vi "0_PlanVirtualStave.vi"(0 "Tape Type":T1=enum."Left stereo", 2 "Stave Locking Points [mm]":dbl[][](array[numeric])=[[0.0, 0.0, 0.0], [280.05, 0.0, 0.0], [574.05, 0.0, 0.0], [868.05, 0.0, 0.0], [1162.05, 0.0, 0.0]], 3 "Code path":path=path "C:/Users/sciollalab/Documents/Brandeis-BNL/LabVIEW_Codes/BNL_ThermomechanicalStave", 5 "Module fiducial marker":T3, 7 "Sensor Pattern":T2=enum."ATLAS12", 9 "N Modules":i32=13, 11 "Working height [mm]":dbl, 12 "error in (no error)":errorcluster, 13 "Stereo Angle [mrad]":dbl=26.0 format="%#_13g") -> (4 "Stave Basis: Coordinates of Fiducials on Modules":dbl[][](array[numeric])=[[-7.689999999999998, -113.212, 0.0], [87.79, -113.212, 0.0], [87.79, -16.13199999999999, 0.0], [-7.689999999999998, -16.13199999999999, 0.0], [90.31, -113.212, 0.0], [185.79000000000002, -113.212, 0.0], [185.79000000000002, -16.13199999999999, 0.0], [90.31, -16.13199999999999, 0.0], [188.31, -113.212, 0.0], [283.79, -113.212, 0.0], [283.79, -16.13199999999999, 0.0], [188.31, -16.13199999999999, 0.0], [286.31, -113.212, 0.0], [381.79, -113.212, 0.0], [381.79, -16.13199999999999, 0.0], [286.31, -16.13199999999999, 0.0], [384.31, -113.212, 0.0], [479.79, -113.212, 0.0], [479.79, -16.13199999999999, 0.0], [384.31, -16.13199999999999, 0.0], [482.30999999999995, -113.212, 0.0], [577.79, -113.212, 0.0], [577.79, -16.13199999999999, 0.0], [482.30999999999995, -16.13199999999999, 0.0], [580.31, -113.212, 0.0], [675.79, -113.212, 0.0], [675.79, -16.13199999999999, 0.0], [580.31, -16.13199999999999, 0.0], [678.31, -113.212, 0.0], [773.79, -113.212, 0.0], [773.79, -16.13199999999999, 0.0], [678.31, -16.13199999999999, 0.0], [776.31, -113.212, 0.0], [871.79, -113.212, 0.0], [871.79, -16.13199999999999, 0.0], [776.31, -16.13199999999999, 0.0], [874.31, -113.212, 0.0], [969.79, -113.212, 0.0], [969.79, -16.13199999999999, 0.0], [874.31, -16.13199999999999, 0.0], [972.31, -113.212, 0.0], [1067.79, -113.212, 0.0], [1067.79, -16.13199999999999, 0.0], [972.31, -16.13199999999999, 0.0], [1070.31, -113.212, 0.0], [1165.79, -113.212, 0.0], [1165.79, -16.13199999999999, 0.0], [1070.31, -16.13199999999999, 0.0], [1168.31, -113.212, 0.0], [1263.79, -113.212, 0.0], [1263.79, -16.13199999999999, 0.0], [1168.31, -16.13199999999999, 0.0]], 14 "error out":errorcluster, 15 "Module fiducials in the Stave's basis":T4(graph)=[{"Generated List of Module Coordinates"=[0.0, 280.05, 574.05, 868.05, 1162.05], "Generated List of Module Coordinates"=[0.0, 0.0, 0.0, 0.0, 0.0]}, {"Generated List of Module Coordinates"=[-7.689999999999998, 87.79, 87.79, -7.689999999999998, 90.31, 185.79000000000002, 185.79000000000002, 90.31, 188.31, 283.79, 283.79, 188.31, 286.31, 381.79, 381.79, 286.31, 384.31, 479.79, 479.79, 384.31, 482.30999999999995, 577.79, 577.79, 482.30999999999995, 580.31, 675.79, 675.79, 580.31, 678.31, 773.79, 773.79, 678.31, 776.31, 871.79, 871.79, 776.31, 874.31, 969.79, 969.79, 874.31, 972.31, 1067.79, 1067.79, 972.31, 1070.31, 1165.79, 1165.79, 1070.31, 1168.31, 1263.79, 1263.79, 1168.31], "Generated List of Module Coordinates"=[-113.212, -113.212, -16.13199999999999, -16.13199999999999, -113.212, -113.212, -16.13199999999999, -16.13199999999999, -113.212, -113.212, -16.13199999999999, -16.13199999999999, -113.212, -113.212, -16.13199999999999, -16.13199999999999, -113.212, -113.212, -16.13199999999999, -16.13199999999999, -113.212, -113.212, -16.13199999999999, -16.13199999999999, -113.212, -113.212, -16.13199999999999, -16.13199999999999, -113.212, -113.212, -16.13199999999999, -16.13199999999999, -113.212, -113.212, -16.13199999999999, -16.13199999999999, -113.212, -113.212, -16.13199999999999, -16.13199999999999, -113.212, -113.212, -16.13199999999999, -16.13199999999999, -113.212, -113.212, -16.13199999999999, -16.13199999999999, -113.212, -113.212, -16.13199999999999, -16.13199999999999]}, {"Generated List of Module Coordinates"=[40.050000000000004, 138.05, 236.05, 334.05, 432.05, 530.05, 628.05, 726.05, 824.05, 922.05, 1020.05, 1118.05, 1216.05], "Generated List of Module Coordinates"=[-64.672, -64.672, -64.672, -64.672, -64.672, -64.672, -64.672, -64.672, -64.672, -64.672, -64.672, -64.672, -64.672]}])   [LabVIEW 2016]
uses:
  Utils/Controls/All_Enums/Enum_TypeDef_FidMarkers.ctl
  Utils/Controls/All_Enums/Enum_TypeDef_Sensors.ctl
  Utils/Controls/All_Enums/Enum_TypeDef_TapeType.ctl
panel:
  in  "Intermodule pitch [mm]":dbl=98.0
  out "Module height [mm]":dbl=97.54
  out "Module width [mm]":dbl=97.54
  in  "Tab Control":enum32{"Stave Configuration", "Error reporting"}(tab)
  out "Stave orientation":bool=TRUE
  in  "Module centre [mm]":T5
  # "PLAN VIRTUAL STAVE Brandeis University - Brookhaven National Laboratory * ATLAS Phase II Inner Tracker Upgrade"
  # "F"
  # "F"
  # "F"
  # "F"
  # "This VI calculates the positions of all fiducials, \"F\",  on the modules on the stave. Supply the bus tape type, sensor design, desired fiducial marker, and number of modules."
  # "F"
  # "F"
  # "F"
  # "F"
  # "Provided by Camera Calibration:"
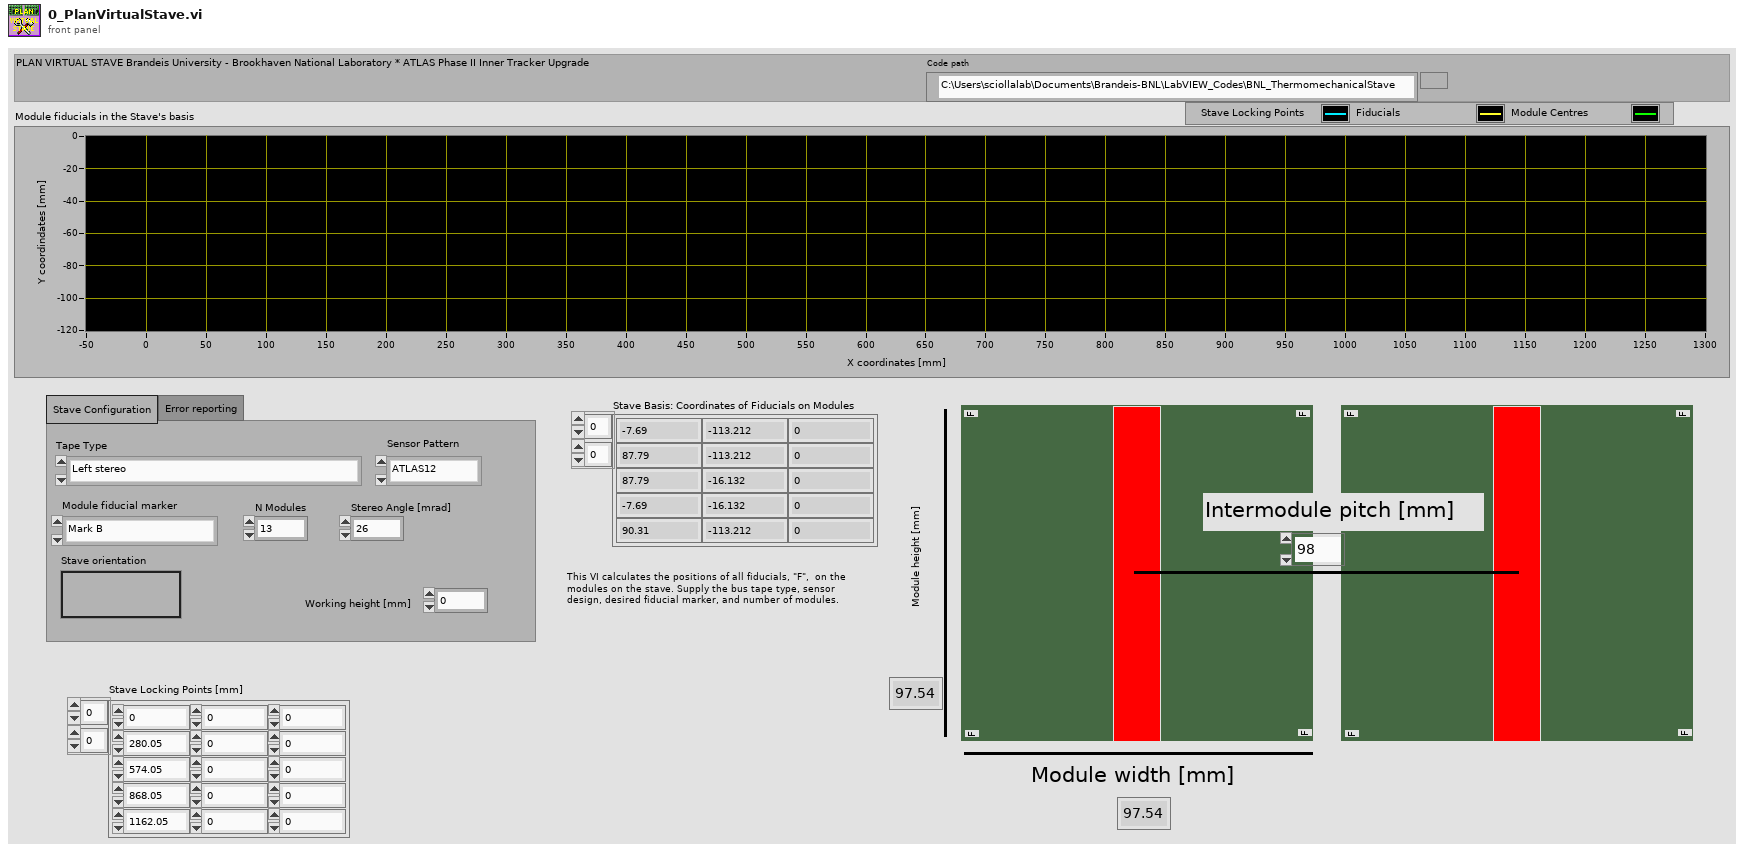
[diagram p1: front panel]
types:
  T1 = typedef "Enum_TypeDef_TapeType.ctl" = enum16{"Right stereo", "Left stereo", "Stereo (Sutcliffe NP49-01-100 01-Mar-16)", "Axial (Sutcliffe NP49-01-100 01-Mar-16)"}
  T2 = typedef "Enum_TypeDef_Sensors.ctl" = enum16{"ATLAS07", "ATLAS12", "ATLAS12Slim", "ATLAS17LS"}
  T3 = typedef "Enum_TypeDef_FidMarkers.ctl" = enum16{"Mark B", "Mark C", "Bias Ring Corner", "Mark I (Slim/17)", "Mark E (Slim/17)", "Mark F (Slim/17)", "Mark G (Slim/17)", "Mark A (12)", "Kapton Spacers"}
  T4 = cluster{"Generated List of Module Coordinates":dbl[], "Generated List of Module Coordinates":dbl[]}[]
  T5 = cluster{"X [mm]":dbl, "Y [mm]":dbl, "Z [mm]":dbl}
  T6 = enum8{"Enabled", "Disabled", "Disabled and Grayed Out"}
  T7 = cluster{"Stave Locking Points [mm]":dbl[], "Stave Locking Points [mm]":dbl[]}
  T8 = cluster{"Generated List of Module Coordinates":dbl[], "Generated List of Module Coordinates":dbl[]}
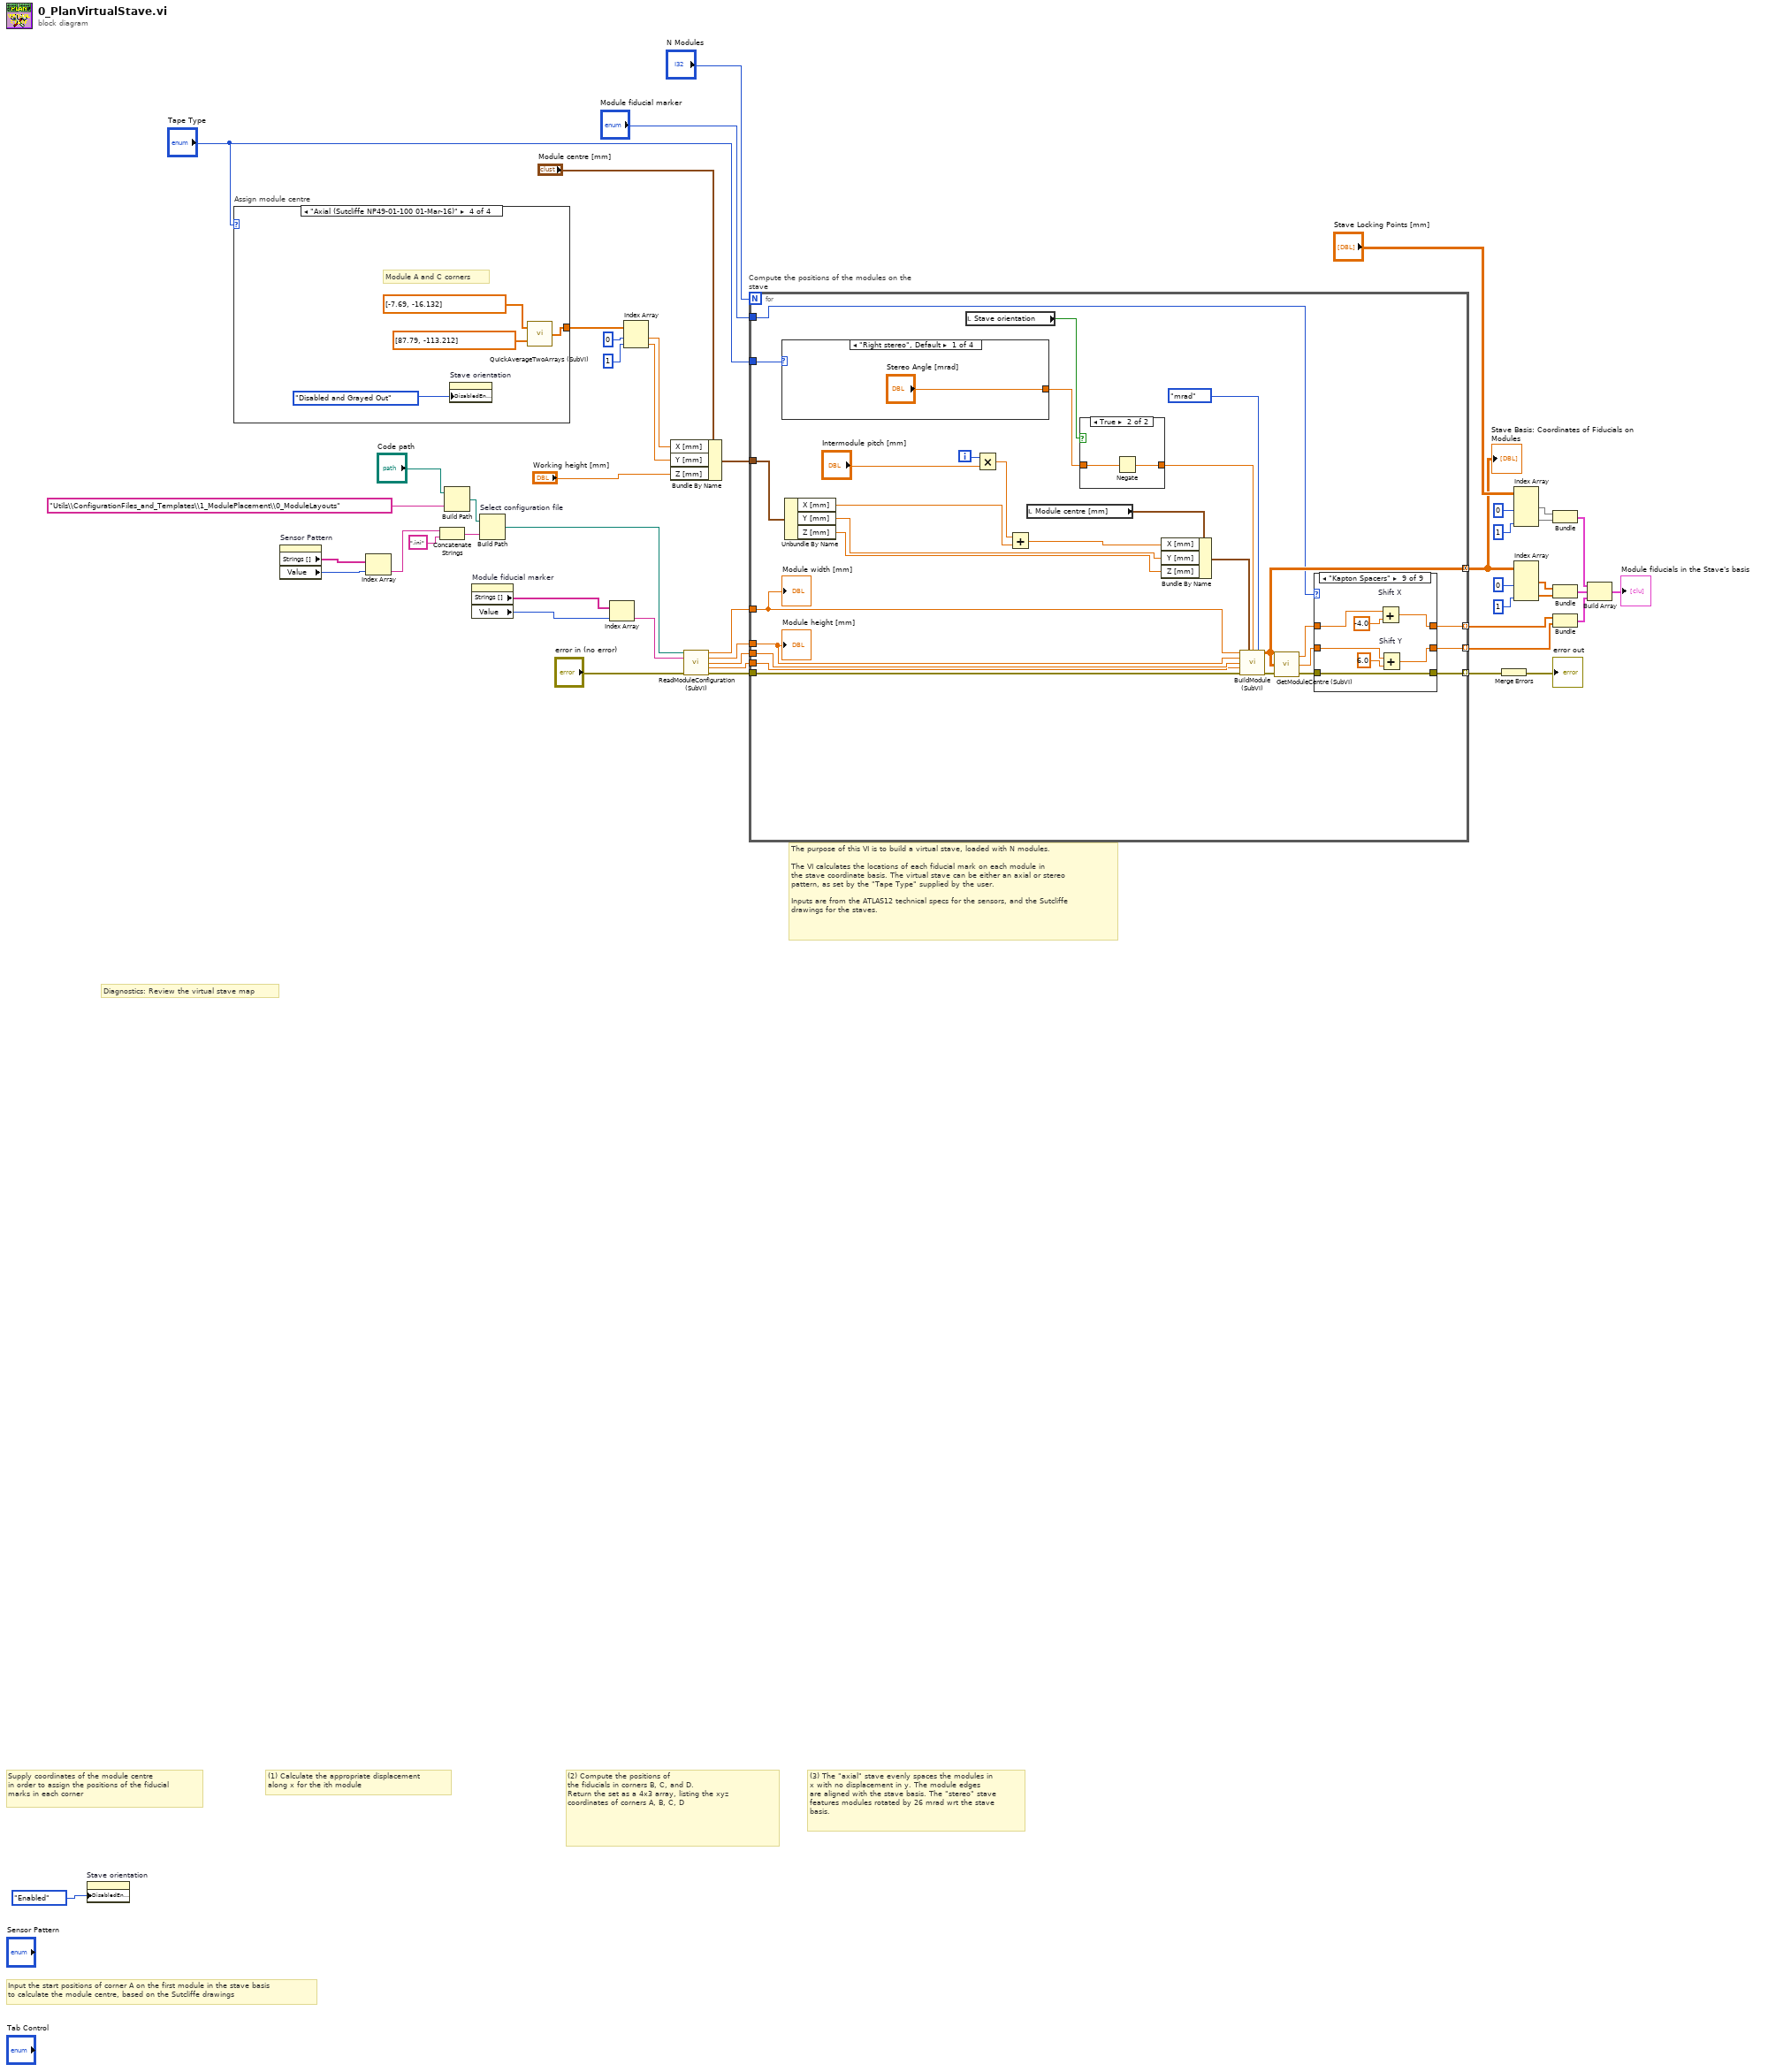
[diagram p0: block diagram]
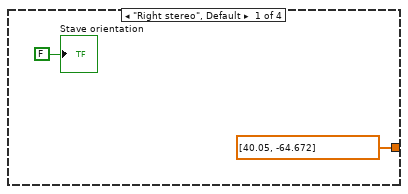
[diagram p2: hidden frame]
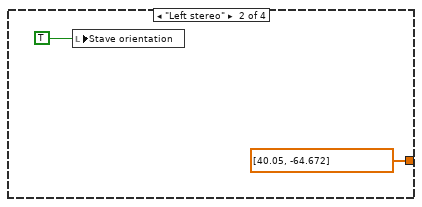
[diagram p3: hidden frame]
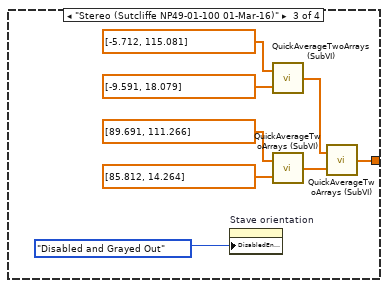
[diagram p4: hidden frame]
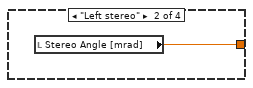
[diagram p14: hidden frame]
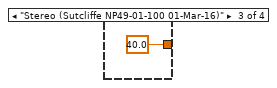
[diagram p15: hidden frame]
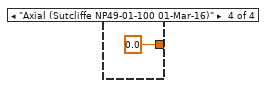
[diagram p16: hidden frame]
diagram:
  # "(1) Calculate the appropriate displacement \nalong x for the ith module"
  # "(3) The \"axial\" stave evenly spaces the modules in \nx with no displacement in y. The module edges \nare aligned with the stave basis. The \"stereo\" stave \nfeatures modules rotated by 26 mrad wrt the stave\nbasis."
  # "(2) Compute the positions of \nthe fiducials in corners B, C, and D. \nReturn the set as a 4x3 array, listing the xyz coordinates of corners A, B, C, D"
  # "Supply coordinates of the module centre \nin order to assign the positions of the fiducial \nmarks in each corner"
  # "Diagnostics: Review the virtual stave map"
  # "Input the start positions of corner A on the first module in the stave basis\nto calculate the module centre, based on the Sutcliffe drawings"
  # "The purpose of this VI is to build a virtual stave, loaded with N modules.\n\nThe VI calculates the locations of each fiducial mark on each module in \nthe stave coordinate basis. The virtual stave can be either an axial or stereo \npattern, as set by the \"Tape Type\" supplied by the user.\n\nInputs are from the ATLAS12 technical specs for the sensors, and the Sutcliffe\ndrawings for the staves."
  n1 = property on="Stave orientation" class="Bool"("DisabledEnum"=T6."Enabled" ("Disabled")) -> ()  [unwired: 2 in, 2 out]
  n2 = case "Assign module centre" shown="\"Axial (Sutcliffe NP49-01-100 01-Mar-16)\"" "Tape Type" {
    tunnel: [dbl[] [40.05, -64.672] ("Average of A and B") dbl[] [40.05, -64.672] ("Average of A and B") w54 w62] -> w27
    frame "Right stereo", Default {
      "Stave orientation" <- FALSE ("Stave orientation")
    }
    frame "Left stereo" {
      n3 = local write "Stave orientation"(TRUE ("Stave orientation")) -> ()
    }
    frame "Stereo (Sutcliffe NP49-01-100 01-Mar-16)" {
      n4 = property on="Stave orientation" class="Bool"("DisabledEnum"=T6."Disabled and Grayed Out" ("Disabled")) -> ()  [unwired: 2 in, 2 out]
      n5 = call "QuickAverageTwoArrays (SubVI).vi"("B"=dbl[] [-9.591, 18.079], "A"=dbl[] [-5.712, 115.081]) -> ("Average of A and B"=w59:dbl[])
      n6 = call "QuickAverageTwoArrays (SubVI).vi"("B"=dbl[] [85.812, 14.264], "A"=dbl[] [89.691, 111.266]) -> ("Average of A and B"=w60:dbl[])
      n7 = call "QuickAverageTwoArrays (SubVI).vi"("B"=w60, "A"=w59) -> ("Average of A and B"=w54:dbl[])
    }
    frame "Axial (Sutcliffe NP49-01-100 01-Mar-16)" {
      # "Module A and C corners"
      n8 = property on="Stave orientation" class="Bool"("DisabledEnum"=T6."Disabled and Grayed Out" ("Disabled")) -> ()  [unwired: 2 in, 2 out]
      n9 = call "QuickAverageTwoArrays (SubVI).vi"("B"=dbl[] [87.79, -113.212], "A"=dbl[] [-7.69, -16.132]) -> ("Average of A and B"=w62:dbl[])
    }
  }
  n10 = property on="Sensor Pattern" class="Enum (strict)"() -> ("Strings []"=w7:string[], "Value"=w6:T2)  [unwired: 2 in, 2 out]
  n11 = Index Array(array=w7, index=w6) -> (element=w5:string)
  n12 = Concatenate Strings(w5, ".ini" ("string")) -> (w3:string)
  n13 = Build Path(base path="Code path", name or relative path="Utils\\ConfigurationFiles_and_Templates\\1_ModulePlacement\\0_ModuleLayouts") -> (appended path=w2:path)
  n14 = property on="Module fiducial marker" class="Enum (strict)"() -> ("Strings []"=w10:string[], "Value"=w9:T3)  [unwired: 2 in, 2 out]
  n15 = Build Path "Select configuration file"(base path=w2, name or relative path=w3) -> (appended path=w1:path)
  n16 = Index Array(array=w10, index=w9) -> (element=w8:string)
  n17 = Index Array(array=w27, index #1=0 ("index"), index #2=1 ("index")) -> (element #1=w30:dbl, element #2=w28:dbl)
  n18 = Bundle By Name(cluster="Module centre [mm]", "X [mm]"=w30, "Y [mm]"=w28, "Z [mm]"="Working height [mm]") -> (w44:T5)
  n19 = call "ReadModuleConfiguration (SubVI).vi"("Module configuration file path"=w1, "Fiducial Mark"=w8, "error in (no error)"="error in (no error)") -> ("Width [mm]"=w18:dbl, "Height [mm]"=w17:dbl, "Lx"=w16:dbl, "Ly"=w15:dbl, "error out"=w19:errorcluster)  [unwired: 6 in, 2 out]
  n20 = for "Compute the positions of the modules on the stave" {
    N: "N Modules" -> [_]
    tunnel: w44 -> [w87]
    tunnel: [w84] -> w12 mode=concatenating
    tunnel: [w70] -> w36 mode=indexing
    tunnel: [w68] -> w26 mode=indexing
    tunnel: [w66] -> w24 mode=indexing
    tunnel: w19 -> [w82]
    tunnel: w18 -> [w79]
    tunnel: w17 -> [w78]
    tunnel: w16 -> [w81]
    tunnel: w15 -> [w80]
    tunnel: "Tape Type" -> [w75]
    tunnel: "Module fiducial marker" -> [w65]
    i -> [w93]
    n21 = case shown="\"Right stereo\", Default" w75 {
      tunnel: ["Stereo Angle [mrad]" w129 40.0 ("Stereo Angle [mrad]") 0.0 ("Angle")] -> w73
      frame "Right stereo", Default {
      }
      frame "Left stereo" {
        n22 = local read "Stereo Angle [mrad]"() -> (w129:dbl)
      }
      frame "Stereo (Sutcliffe NP49-01-100 01-Mar-16)" {
      }
      frame "Axial (Sutcliffe NP49-01-100 01-Mar-16)" {
      }
    }
    n23 = Unbundle By Name(w87) -> ("X [mm]"=w92:dbl, "Y [mm]"=w90:dbl, "Z [mm]"=w88:dbl)
    n24 = local read "Stave orientation"() -> (w74:bool)
    n25 = Multiply(x=w93, y="Intermodule pitch [mm]") -> (x*y=w91:dbl)
    n26 = Add(x=w91, y=w92) -> (x+y=w89:dbl)
    n27 = local read "Module centre [mm]"() -> (w76:T5)
    n28 = case shown="True" w74 {
      tunnel: w73 -> [w125 w127]
      tunnel: [w125 w126] -> w72
      frame False {
      }
      frame True {
        n29 = Negate(x=w127) -> (-x=w126:dbl)
      }
    }
    n30 = Bundle By Name(cluster=w76, "X [mm]"=w89, "Y [mm]"=w90, "Z [mm]"=w88) -> (w86:T5)
    n31 = call "BuildModule (SubVI).vi"("Module width[mm]"=w79, "Module Centre [mm]"=w86, "Angle"=w72, "Units"=enum16{"mrad", "Radians", "Degrees"}."mrad", "Module height [mm]"=w78, "x to fiducial [um]"=w81, "y to fiducial [um]"=w80, "error in (no error)"=w82) -> ("Generated List of Module Coordinates"=w84:dbl[][], "error out"=w83:errorcluster)  [unwired: 6 in]
    n32 = call "GetModuleCentre (SubVI).vi"("error in (no error)"=w83, "4x3 Array of Fiducial Coordinates"=w84) -> ("error out"=w67:errorcluster, "y, centre"=w69:dbl, "x, centre"=w71:dbl)  [unwired: 1 in]
    n33 = case shown="\"Kapton Spacers\"" w65 {
      tunnel: w71 -> [w96 w99 w101 w105 w107 w110 w113 w117 w121]
      tunnel: [w96 w99 w101 w105 w107 w110 w113 w117 w120] -> w70
      tunnel: w69 -> [w95 w98 w100 w104 w106 w109 w112 w116 w124]
      tunnel: [w95 w98 w100 w104 w106 w109 w112 w116 w119] -> w68
      tunnel: w67 -> [w94 w97 w102 w103 w108 w111 w114 w115 w118]
      tunnel: [w94 w97 w102 w103 w108 w111 w114 w115 w118] -> w66
      frame "Mark B", Default {
      }
      frame "Mark C" {
      }
      frame "Bias Ring Corner" {
      }
      frame "Mark I (Slim/17)" {
      }
      frame "Mark E (Slim/17)" {
      }
      frame "Mark F (Slim/17)" {
      }
      frame "Mark G (Slim/17)" {
      }
      frame "Mark A (12)" {
      }
      frame "Kapton Spacers" {
        n34 = Add "Shift X"(x=w121, y=-4.0) -> (x+y=w120:dbl)
        n35 = Add "Shift Y"(x=w124, y=6.0) -> (x+y=w119:dbl)
      }
    }
    "Module width [mm]" <- w79
    "Module height [mm]" <- w78
  }
  "Stave Basis: Coordinates of Fiducials on Modules" <- w12
  n36 = Merge Errors(w24) -> (→"error out":errorcluster)
  n37 = Index Array(array="Stave Locking Points [mm]", index (col) #1=0 ("disabled index (col)"), index (col) #2=1 ("disabled index (col)")) -> (element #1=w40:dbl[], element #2=w39:dbl[])  [unwired: 2 in]
  n38 = Index Array(array=w12, index (col) #1=0 ("disabled index (col)"), index (col) #2=1 ("index (col)")) -> (element #1=w48:dbl[], element #2=w47:dbl[])  [unwired: 2 in]
  n39 = Bundle("Stave Locking Points [mm]"=w40, "Stave Locking Points [mm]"=w39) -> (w33:T7)  [unwired: 1 in]
  n40 = Bundle("Generated List of Module Coordinates"=w48, "Generated List of Module Coordinates"=w47) -> (w35:T8)  [unwired: 1 in]
  n41 = Bundle(w36, w26) -> (w34:cluster{dbl[], dbl[]})  [unwired: 1 in]
  n42 = Build Array(w33, w35, w34) -> (→"Module fiducials in the Stave's basis":T4)
